vi "Read Window Write Size.vi"(8 "Error In":errorcluster, 11 "Channel In":refnum<class "Channel.lvclass">) -> (0 "Error Out":errorcluster, 2 "Write Size":u32, 3 "Channel Out":refnum<class "Channel.lvclass">)   [LabVIEW 2021, in "Field_RnD_Services_LIBSSH2_Toolkit.lvlib" / "Channel.lvclass"]
doc: "Gets the window write size in bytes (B)."
uses:
  Channel.lvclass
  Session/Session.lvclass
  Field_RnD_Services_LIBSSH2_Toolkit.lvlib
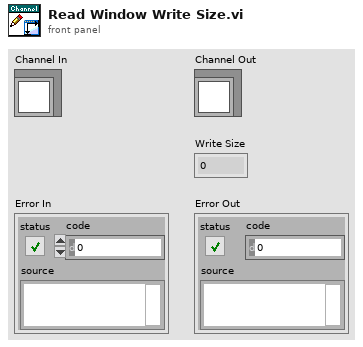
[diagram p1: front panel]
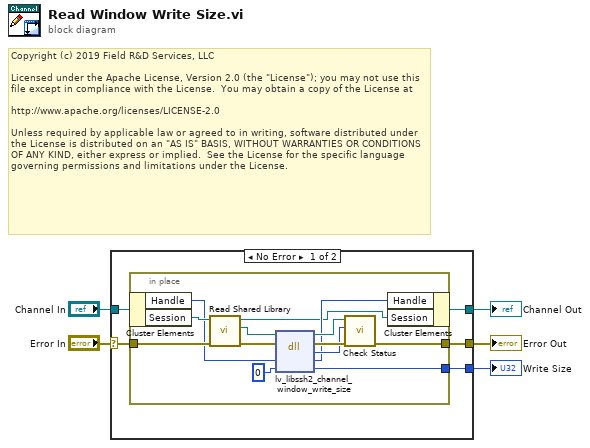
[diagram p0: block diagram]
diagram:
  # "Copyright (c) 2019 Field R&D Services, LLC\n\nLicensed under the Apache License, Version 2.0 (the \"License\"); you may not use this file except in compliance with the License.  You may obtain a copy of the License at\n\nhttp://www.apache.org/licenses/LICENSE-2.0\n\nUnless required by applicable law or agreed to in writing, software distributed under the License is distributed on an \"AS IS\" BASIS, WITHOUT WARRANTIES OR CONDITIONS OF ANY KIND, either express or implied.  See the License for the specific language governing permissions and limitations under the License."
  n1 = case shown="No Error" "Error In" {
    selector: "Error In" -> [w8 w25]
    tunnel: [w7 w25] -> w4
    tunnel: "Channel In" -> [w10 w24]
    tunnel: [w9 w24] -> w2
    tunnel: [w6 _] -> w1
    frame No Error {
      n2 = in-place {
        in-place-border: w8 -> [w21]
        in-place-border: [w17] -> w7
        in-place-border: [w11] -> w6
        n3 = in-place-cluster #1(w10) -> ("Handle"=w16:u64, "Session"=w23:refnum<class "Session.lvclass">)
        n4 = call "Read Shared Library.vi"("Error In"=w21, "Session In"=w23) -> ("Erorr Out"=w13:errorcluster, "libssh2lv Shared Library"=w22:path, "Session Out"=w14:refnum<class "Session.lvclass">)  [unwired: 7 in]
        n5 = dll-call lib="libssh2lv.*" fn="lv_libssh2_channel_window_write_size"(path in=w22, error in=w13, "handle"=w16, "size"=u32 0) -> (path out=w19:path, error out=w20:errorcluster, "status"=w18:i32, "handle"=w15:u64, "size"=w11:u32)  [unwired: 1 in]
        n6 = call "Check Status.vi"("Error In"=w20, "Status"=w18, "libssh2lv Shared Library In"=w19) -> ("Error Out"=w17:errorcluster)  [unwired: 7 in, 1 out]
        n7 = in-place-cluster #1("Handle"=w15, "Session"=w14) -> (w9:refnum<class "Channel.lvclass">)
      }
    }
    frame Error {
    }
  }
  "Error Out" <- w4
  "Channel Out" <- w2
  "Write Size" <- w1
